vi "Populate Enum Strings.vi"(8 "error in (no error)":errorcluster, 10 "Strings []":string[](array[string])=["This", "is", "after"], 11 "Control Path":path=path "enum_target.vi") -> (0 "error out":errorcluster)   [LabVIEW 2009]
doc: "Copyright © 2005, Soliton Technologies.\nAll rights reserved."
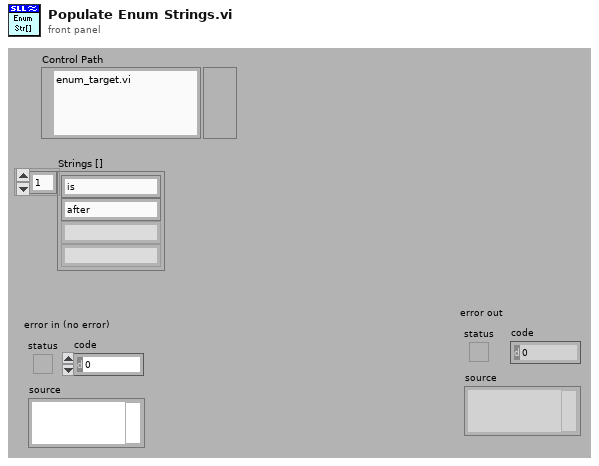
[diagram p1: front panel]
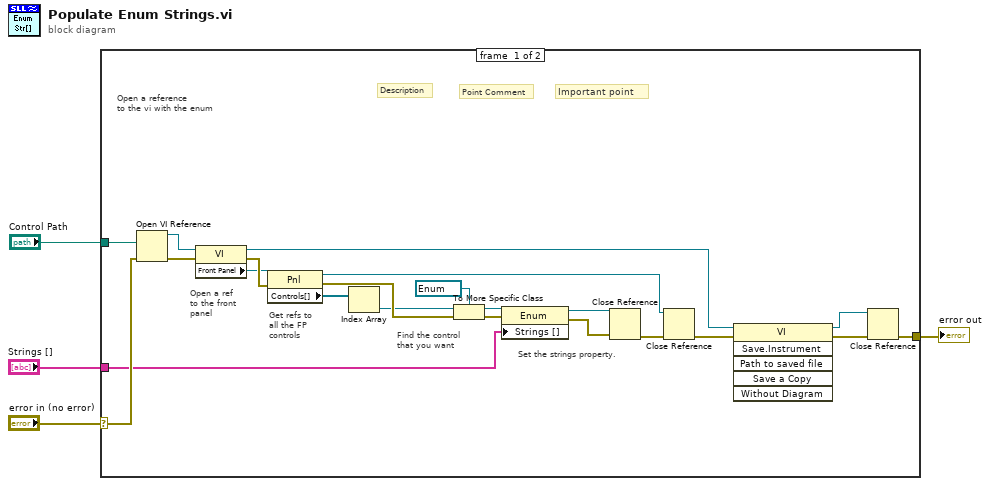
[diagram p0: block diagram]
diagram:
  n1 = case shown="No Error" "error in (no error)" {
    selector: "error in (no error)" -> [w22 w27]
    tunnel: [w21 w27] -> w3
    tunnel: "Control Path" -> [w23 _]
    tunnel: "Strings []" -> [w13 _]
    frame #0 {
      # "Set the strings property."
      # "Find the control\nthat you want"
      # "Get refs to\nall the FP\ncontrols"
      # "Open a ref\nto the front\npanel"
      # "Open a reference\nto the vi with the enum"
      # "Point Comment"
      # "Important point"
      # "Description"
      n2 = Open VI Reference(vi path=w23, error in (no error)=w22) -> (vi reference=w5:refnum<vi>, error out=w26:errorcluster)  [unwired: 4 in]
      n3 = property class="VI"(reference=w5, error in=w26) -> (reference out=w12:refnum<vi>, error out=w25:errorcluster, "Front Panel"=w6:refnum<vi>)
      n4 = property class="Pnl"(reference=w6, error in=w25) -> (reference out=w7:refnum<vi>, error out=w15:errorcluster, "Controls[]"=w20:refnum<vi>[])
      n5 = Index Array(array=w20) -> (element=w8:refnum<vi>)  [unwired: 1 in]
      n6 = To More Specific Class(target class=refnum<vi> refnum, reference=w8, error in=w15) -> (specific class reference=w19:refnum<vi>, error out=w17:errorcluster)
      n7 = property class="Enum"(reference=w19, error in=w17, "Strings []"=w13) -> (reference out=w18:refnum<vi>, error out=w16:errorcluster)
      n8 = Close Reference(reference=w18, error in (no error)=w16) -> (error out=w24:errorcluster)
      n9 = Close Reference(reference=w7, error in (no error)=w24) -> (error out=w11:errorcluster)
      n10 = invoke class="VI" method="Save.Instrument"(reference=w12, error in=w11) -> (reference out=w9:refnum<vi>, error out=w10:errorcluster)  [unwired: 4 in, 4 out]
      n11 = Close Reference(reference=w9, error in (no error)=w10) -> (error out=w21:errorcluster)
    }
    frame #1 {
    }
  }
  "error out" <- w3
